vi "Configure Continuous Generation.vi"(0 "RFSG handle":refnum<k15>, 5 "Waveform in":T1 {"Runtime Scaling" format="%#_6p"; "Sample Rate" format="%#_6p"; "Burst Length (s)" format="%#_6p"; "PAPR (dB)" format="%.2f"; "Signal Bandwidth (Hz)" format="%#_6p"}, 7 "Waveform Start Trigger Export":T2="PXI_Trig0", 11 "error in":errorcluster) -> (4 "RFSG handle out":refnum<k15>, 6 "Waveform out":T1 {"Runtime Scaling" format="%#_6p"; "Sample Rate" format="%#_6p"; "Burst Length (s)" format="%#_6p"; "PAPR (dB)" format="%.2f"; "Signal Bandwidth (Hz)" format="%#_6p"}, 15 "error out":errorcluster)   [LabVIEW 2016, in "SG.lvlib"]
doc: "Configures the generator to generate the waveform continuously with a trigger on the first sample of the waveform. Use <b>Abort Generation</b> to abort generation to always ensure complete packet generation."
uses:
  SG.lvlib
  Common/Waveform.ctl
  <instrlib>/niRFSG/niRFSG.llb/niRFSG Exported Signal Destinations.ctl
  <instrlib>/niRFSG/niRFSG.llb/niRFSG Signal Names.ctl
  <instrlib>/niRFSG/niRFSG.llb/niRFSG Signal Identifiers.ctl
  <instrlib>/niRFSG/niRFSG.llb/niRFSG Script Trigger IDs.ctl
  <instrlib>/niRFSG/niRFSG.llb/niRFSG Configure Script Trigger Software.vi
  Common/Common.lvlib
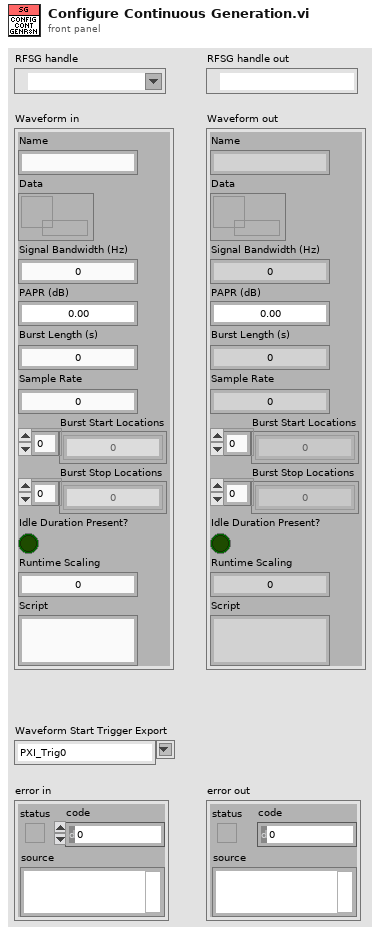
[diagram p1: front panel]
types:
  T1 = typedef "Common.lvlib/Waveform.ctl" = cluster{"Name":string, "Data":refnum<data-value>, "Signal Bandwidth (Hz)":dbl, "PAPR (dB)":dbl, "Burst Length (s)":dbl, "Sample Rate":dbl, "Burst Start Locations":i32[], "Burst Stop Locations":i32[], "Idle Duration Present?":bool, "Runtime Scaling":dbl, "Script":string}
  T2 = typedef "niRFSG Exported Signal Destinations.ctl" = string
  T3 = typedef "niRFSG Script Trigger IDs.ctl" = string
  T4 = typedef "niRFSG Signal Identifiers.ctl" = string
  T5 = typedef "niRFSG Signal Names.ctl" = i32
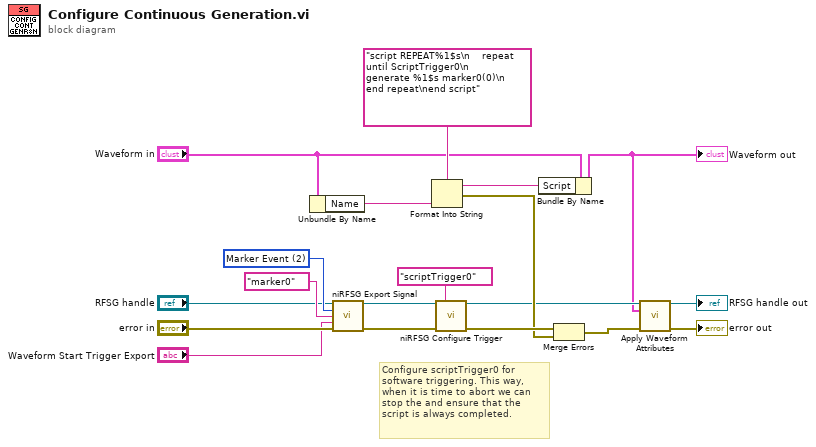
[diagram p0: block diagram]
diagram:
  w13 = T5 2 items=["Start Trigger", "Script Trigger", "Marker Event", "Ref Clock", "Started Event", "Done Event", "Configuration List Step Trigger", "Configuration Settled Event"] ("signal")
  # "Configure scriptTrigger0 for software triggering. This way, when it is time to abort we can stop the and ensure that the script is always completed."
  n1 = Unbundle By Name("Waveform in") -> ("Name"=w6:string)
  n2 = call <instrlib>:"niRFSG Export Signal.vi"("instrument handle"="RFSG handle", "signal"=w13, "signal identifier"=T4 "marker0", "output terminal"="Waveform Start Trigger Export", "error in"="error in") -> ("instrument handle out"=w10:refnum<k15>, "error out"=w16:errorcluster)  [unwired: 9 in]
  n3 = Format Into String(format string="script REPEAT%1$s\n    repeat until ScriptTrigger0\n        generate %1$s marker0(0)\n    end repeat\nend script", w6) -> (resulting string=w1:string, error out=w14:errorcluster)  [unwired: 2 in]
  n4 = call-poly <instrlib>:"niRFSG Configure Trigger.vi"("instrument handle"=w10, "trigger id"=T3 "scriptTrigger0", "error in"=w16) -> ("instrument handle out"=w4:refnum<k15>, "error out"=w17:errorcluster)  [unwired: 11 in]
  n5 = Bundle By Name(cluster="Waveform in", "Script"=w1) -> (w2:T1)
  "Waveform out" <- w2
  n6 = Merge Errors(w17, w14) -> (w15:errorcluster)
  n7 = call "Apply Waveform Attributes.vi"("RFSG Session In"=w4, "Waveform"=w2, "error in (no error)"=w15) -> ("RFSG Session Out"=→"RFSG handle out":refnum<k15>, "error out"=→"error out":errorcluster)  [unwired: 11 in]
